vi "Flush.vi"(8 "Error In":errorcluster) -> (0 "Error Out":errorcluster, 2 "No. Of Remaining Elements":i32, 3 "Remaining Elements":T1[](array[typedef]))   [LabVIEW 2023, in "Error Manager.lvlib" / "MHL Queue.lvlib"]
doc: "Flushes (dequeues) all the elements from the queue. The queue is empty immediately after this VI executes."
uses:
  MHL Queue.lvlib
  Message (cluster).ctl
  Command (enum).ctl
  Queue Reference (library variable).vi
panel:
  # "Input\nInputs to the VI"
  # "Development\nControls or indicators that are useful for development or testing, but which are not outputs of the VI."
  # "Output\nOutputs of the VI"
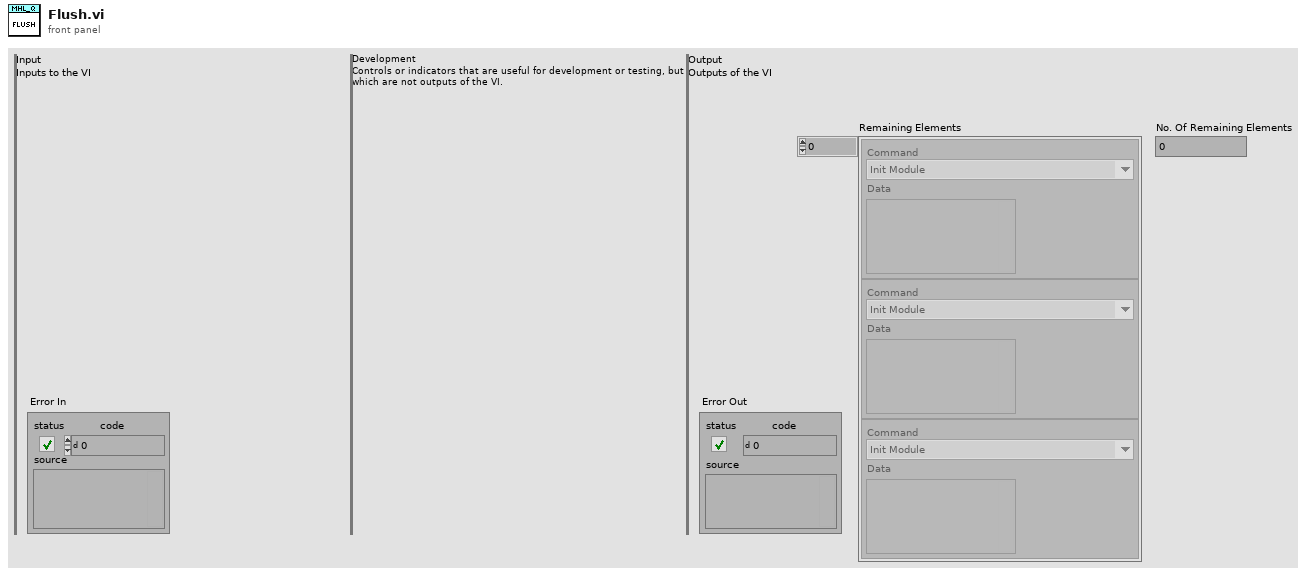
[diagram p1: front panel]
types:
  T1 = typedef "Error Manager.lvlib/MHL Queue.lvlib/Message (cluster).ctl" = cluster{"Command":T2, "Data":variant}
  T2 = typedef "Error Manager.lvlib/MHL Queue.lvlib/Command (enum).ctl" = enum16{"Init Module", "Close Module", "Internal Error", "Create Error Log File", "Show Front Panel", "Handle Error", "Refresh MCL", "MCL Value Change", "Mark Error As Read", "Mark All Errors As Read", "Change Display Order", "One-Second Interval Expired"}
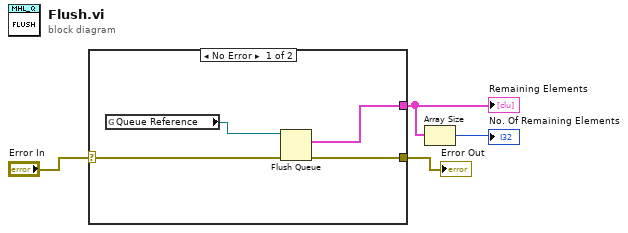
[diagram p0: block diagram]
diagram:
  n1 = case shown="No Error" "Error In" {
    selector: "Error In" -> [w7 w9]
    tunnel: [w8 w9] -> w3
    tunnel: [w6 _] -> w2
    frame No Error {
      n2 = global read "Queue Reference (library variable).vi" "Queue Reference"() -> (w5:refnum<queue>)
      n3 = Flush Queue(queue=w5, error in (no error)=w7) -> (remaining elements=w6:T1[], error out=w8:errorcluster)  [unwired: 1 out]
    }
    frame Error {
    }
  }
  "Error Out" <- w3
  "Remaining Elements" <- w2
  n4 = Array Size(array=w2) -> (size(s)=→"No. Of Remaining Elements":i32)
